vi "CalcUIControl.vi"(6 "warn_limit":dbl, 7 "err_limit":dbl, 9 "curr_val":dbl, 10 "event":string, 11 "PredictiveMaintenance in":refnum<class "PredictiveMaintenance.lvclass">) -> (3 "UICtrl_Data":T1 {"slider_background" scale=0.0..100.0; "slider" scale=0.0..100.0})   [LabVIEW 2019, in "PredictiveMaintenance.lvlib" / "PredictiveMaintenance.lvclass"]
uses:
  PredictiveMaintenance.lvclass
  typedefs/UI_Control.ctl
  PredictiveMaintenance.lvclass/PredictiveMaintenance.ctl
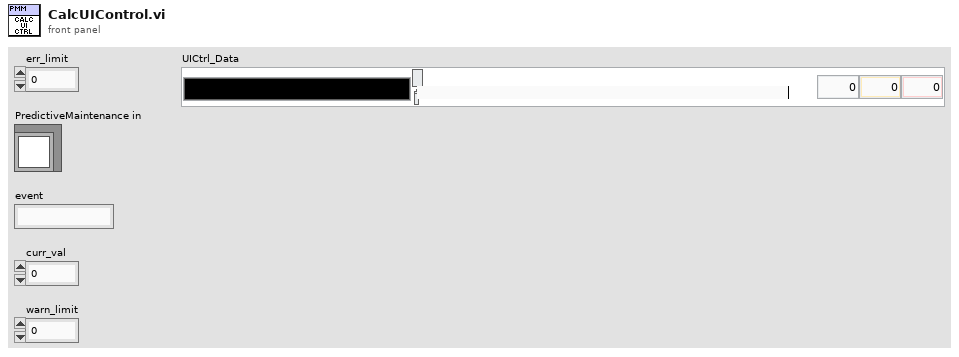
[diagram p1: front panel]
types:
  T1 = typedef "PredictiveMaintenance.lvlib/PredictiveMaintenance.lvclass/UI_Control.ctl" = cluster{"String":string, "slider":dbl, "slider_background":cluster{"Numeric":dbl, "Numeric":dbl, "Numeric":dbl}, "curr_value":dbl, "warn_value":dbl, "err_value":dbl, "colorbox":u32}
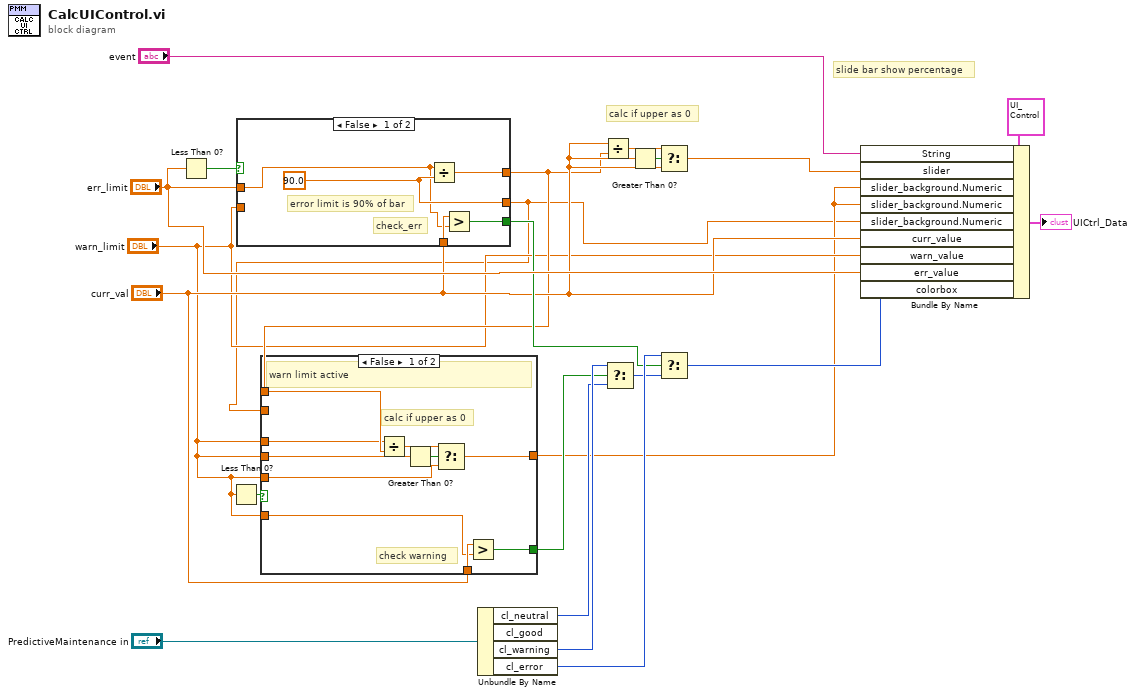
[diagram p0: block diagram]
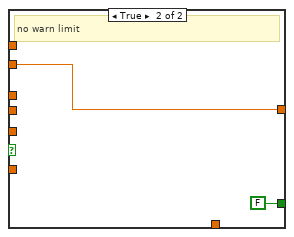
[diagram p2: hidden frame]
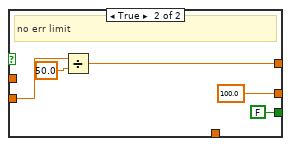
[diagram p3: hidden frame]
diagram:
  # "calc if upper as 0"
  # "slide bar show percentage"
  n1 = Less Than 0?(x="err_limit") -> (x < 0?=w18:bool)
  n2 = Less Than 0?(x="warn_limit") -> (x < 0?=w5:bool)
  n3 = case shown="False" w18 {
    tunnel: [w27 100.0 ("y")] -> w1
    tunnel: [w26 w29] -> w4
    tunnel: "err_limit" -> [w23 _]
    tunnel: "warn_limit" -> [_ w31]
    tunnel: "curr_val" -> [w25 _]
    tunnel: [w24 FALSE] -> w8
    frame False {
      w27 = 90.0 ("y")
      # "check_err"
      # "error limit is 90% of bar"
      n4 = Divide(x=w23, y=w27) -> (x/y=w26:dbl)
      n5 = Greater?(x=w25, y=w23) -> (0:w24:bool)
    }
    frame True {
      # "no err limit"
      n6 = Divide(x=w31, y=50.0) -> (x/y=w29:dbl)
    }
  }
  n7 = case shown="False" w5 {
    tunnel: "warn_limit" -> [w33 _]
    tunnel: "curr_val" -> [w42 _]
    tunnel: [w41 FALSE] -> w6
    tunnel: "warn_limit" -> [w38 _]
    tunnel: "warn_limit" -> [w37 _]
    tunnel: w4 -> [w36 _]
    tunnel: "warn_limit" -> [w35 _]
    tunnel: [w34 w43] -> w2
    tunnel: w1 -> [_ w43]
    frame False {
      # "calc if upper as 0"
      # "check warning"
      # "warn limit active"
      n8 = Divide(x=w35, y=w36) -> (x/y=w39:dbl)
      n9 = Greater Than 0?(x=w37) -> (x > 0?=w40:bool)
      n10 = Select(t=w39, s=w40, f=w38) -> (s? t:f=w34:dbl)
      n11 = Greater?(x=w42, y=w33) -> (0:w41:bool)
    }
    frame True {
      # "no warn limit"
    }
  }
  n12 = Unbundle By Name("PredictiveMaintenance in") -> ("cl_neutral"=w19:u32, "cl_warning"=w20:u32, "cl_error"=w21:u32)  [unwired: 1 out]
  n13 = Divide(x="curr_val", y=w4) -> (x/y=w13:dbl)
  n14 = Select(t=w20, s=w6, f=w19) -> (s? t:f=w15:u32)
  n15 = Greater Than 0?(x="curr_val") -> (x > 0?=w12:bool)
  n16 = Select(t=w13, s=w12, f="curr_val") -> (s? t:f=w14:dbl)
  n17 = Select(t=w21, s=w8, f=w15) -> (s? t:f=w16:u32)
  n18 = Bundle By Name(cluster=T1 {"String"="", "slider"=0.0, "slider_background"={"Numeric"=0.0, "Numeric"=0.0, "Numeric"=0.0}, "curr_value"=0.0, "warn_value"=0.0, "err_value"=0.0, "colorbox"=0} ("Cluster"), "String"="event", "slider"=w14, "slider_background.Numeric"=w2, "slider_background.Numeric"=w2, "slider_background.Numeric"=w1, "curr_value"="curr_val", "warn_value"="warn_limit", "err_value"="err_limit", "colorbox"=w16) -> (→"UICtrl_Data":T1)
